vi "Get Terminal Counts.vi"(8 "error in (no error)":errorcluster, 11 "VI Refnum":refnum<vi>) -> (0 "error out":errorcluster, 3 "Terminal Counts":T1)   [LabVIEW 2018, in "Resource Manipulation.lvlib"]
uses:
  Resource Manipulation.lvlib
  Terminal Counts.ctl
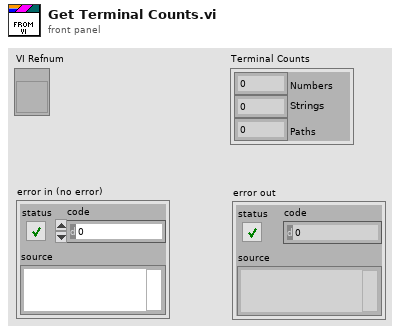
[diagram p1: front panel]
types:
  T1 = typedef "Resource Manipulation.lvlib/Terminal Counts.ctl" = cluster{"Numbers":u32, "Strings":u32, "Paths":u32}
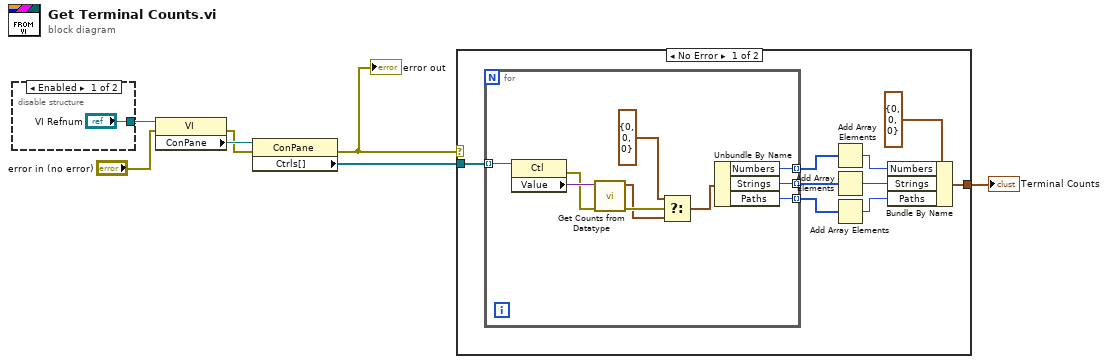
[diagram p0: block diagram]
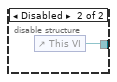
[diagram p3: hidden frame]
diagram:
  n1 = disable-structure shown="Enabled" {
    disable-tunnel: ["VI Refnum" w9] -> w7
    frame Enabled {
    }
    frame Disabled {
      n2 = control-ref of="This VI"() -> (w9:refnum<vi>)
    }
  }
  n3 = property class="VI"(reference=w7, error in="error in (no error)") -> (error out=w3:errorcluster, "ConPane"=w6:refnum<vi>)  [unwired: 1 out]
  n4 = property class="ConPane"(reference=w6, error in=w3) -> (error out=w1:errorcluster, "Ctrls[]"=w5:refnum<vi>[])  [unwired: 1 out]
  "error out" <- w1
  n5 = case shown="No Error" w1 {
    tunnel: w5 -> [w18 _]
    tunnel: [w11 _] -> w2
    frame No Error {
      n6 = for {
        tunnel: w18 -> [w28] mode=indexing
        tunnel: [w25] -> w17 mode=indexing
        tunnel: [w24] -> w16 mode=indexing
        tunnel: [w23] -> w15 mode=indexing
        n7 = property class="Ctl"(reference=w28) -> (error out=w26:errorcluster, "Value"=w27:variant)  [unwired: 1 in, 1 out]
        n8 = call "Get Counts from Datatype.vi"("error in (no error)"=w26, "type"=w27) -> ("error out"=w22:errorcluster, "Terminal Counts"=w21:T1)  [unwired: 8 in]
        n9 = Select(t=T1 {"Numbers"=0, "Strings"=0, "Paths"=0} ("Terminal Counts"), s=w22, f=w21) -> (s? t:f=w20:T1)
        n10 = Unbundle By Name(w20) -> ("Numbers"=w25:u32, "Strings"=w24:u32, "Paths"=w23:u32)
      }
      n11 = Add Array Elements(numeric array=w17) -> (sum=w14:u32)
      n12 = Add Array Elements(numeric array=w16) -> (sum=w13:u32)
      n13 = Add Array Elements(numeric array=w15) -> (sum=w12:u32)
      n14 = Bundle By Name(cluster=T1 {"Numbers"=0, "Strings"=0, "Paths"=0} ("Terminal Counts"), "Numbers"=w14, "Strings"=w13, "Paths"=w12) -> (w11:T1)
    }
    frame Error {
    }
  }
  "Terminal Counts" <- w2
